vi "Tx_UDPoriented.vi"() -> ()   [LabVIEW 2020]
uses:
  AIM664LV.lvlib
  bsp/AFDX_Transmit/Fdx Create Tx VL.vi
  _polimorphicInstances/session/Fdx Create Session (Tx-UDP Port-Oriented).vi
  _polimorphicInstances/control/Fdx Start (Tx).vi
  _polimorphicInstances/control/Fdx Stop (Tx).vi
  _controls/comm_config_vl_tx.ctl
panel:
  out "Duplicated":bool
  out "PortInitOut":T1 {"PortConfig" items=["FDX_SINGLE", "FDX_REDUNDANT"]}
  out "VlId 2":u16
  out "VlId":u16
  out "error out":errorcluster
  in  "VL Config 2":T2={"VlId"=44, "NumOfSubVl"=4, "rate mS (128)"=128.0, "domainID"=2, "sideID"=2, "locationID"=2, "interfaceID"=2, "NetSelect"=3, "Skew"=0, "MaxFrameLength"=1000, "FrameBufferSize"=1000} {"NetSelect" items=["FDX_TX_FRAME_DLY_A"=0, "FDX_TX_FRAME_DLY_B"=1, "FDX_TX_FRAME_BOTH "=3, "FDX_TX_FRAME_ONLY_A"=4, "FDX_TX_FRAME_ONLY_B "=5]; "interfaceID" format="%.0b"}
  in  "VL Config":T2={"VlId"=43, "NumOfSubVl"=4, "rate mS (128)"=128.0, "domainID"=1, "sideID"=1, "locationID"=1, "interfaceID"=1, "NetSelect"=3, "Skew"=0, "MaxFrameLength"=1000, "FrameBufferSize"=1000} {"NetSelect" items=["FDX_TX_FRAME_DLY_A"=0, "FDX_TX_FRAME_DLY_B"=1, "FDX_TX_FRAME_BOTH "=3, "FDX_TX_FRAME_ONLY_A"=4, "FDX_TX_FRAME_ONLY_B "=5]; "interfaceID" format="%.0b"}
  in  "port":u32
  in  "board":u32
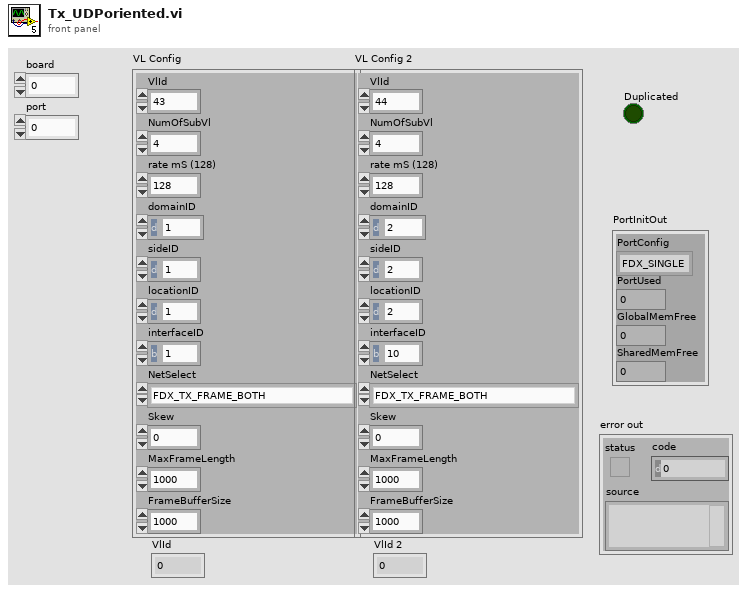
[diagram p1: front panel]
types:
  T1 = cluster{"PortConfig":u32, "PortUsed":u32, "GlobalMemFree":u32, "SharedMemFree":u32}
  T2 = typedef "AIM664LV.lvlib/comm_config_vl_tx.ctl" = cluster{"VlId":u16, "NumOfSubVl":u16, "rate mS (128)":dbl, "domainID":u8, "sideID":u8, "locationID":u8, "interfaceID":u8, "NetSelect":u32, "Skew":u32, "MaxFrameLength":u32, "FrameBufferSize":u32}
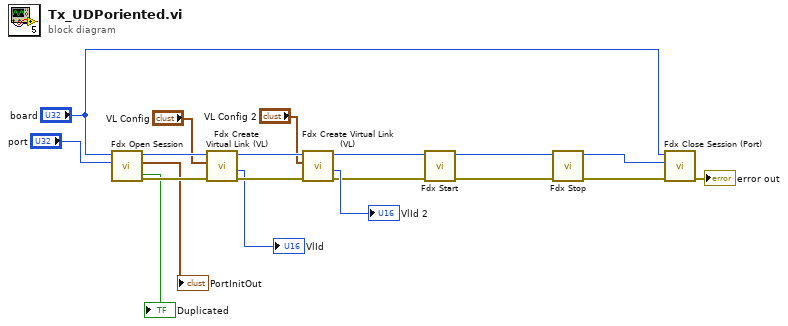
[diagram p0: block diagram]
diagram:
  n1 = call-poly "Fdx Open Session.vi"("port"="port", "board"="board") -> ("error out"=w18:errorcluster, "PortInitOut"=→"PortInitOut":T1, "port handle out"=w19:u32, "Duplicated"=→"Duplicated":bool)  [unwired: 5 in, 1 out]
  n2 = call-poly "Fdx Create Virtual Link (VL).vi"("error in (no error)"=w18, "VL Config"="VL Config", "InstrumentHandle in"=w19) -> ("error out"=w16:errorcluster, "VlId"=→"VlId":u16, "InstrumentHandle out"=w17:u32)  [unwired: 6 in]
  n3 = call-poly "Fdx Create Virtual Link (VL).vi"("error in (no error)"=w16, "VL Config"="VL Config 2", "InstrumentHandle in"=w17) -> ("error out"=w6:errorcluster, "VlId"=→"VlId 2":u16, "InstrumentHandle out"=w7:u32)  [unwired: 6 in]
  n4 = call-poly "Fdx Start.vi"("error in (no error)"=w6, "InstrumentHandle_port in"=w7) -> ("error out"=w4:errorcluster, "InstrumentHandle_port out"=w5:u32)  [unwired: 8 in]
  n5 = call-poly "Fdx Stop.vi"("error in (no error)"=w4, "InstrumentHandle_port in"=w5) -> ("error out"=w3:errorcluster, "InstrumentHandle_port out"=w1:u32)  [unwired: 8 in]
  n6 = call "Fdx Close Session (Port).vi"("error in (no error)"=w3, "InstrumentHandle_port in"=w1, "InstrumentHandle_board in"="board") -> ("error out"=→"error out":errorcluster)  [unwired: 8 in]
